vi "Discrete_TF_L_RT.vi"(10 "Gain":sgl, 11 "Input":sgl format="%#_13g") -> (3 "Output":sgl)   [LabVIEW 2019]
panel:
  in  "Numerator":sgl=5.6754 format="%#_13g"
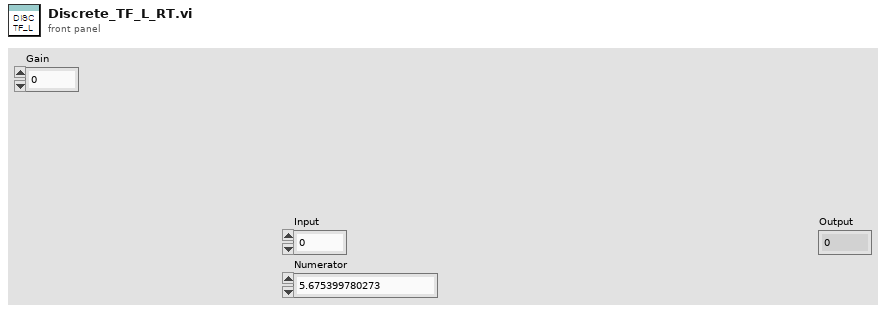
[diagram p1: front panel]
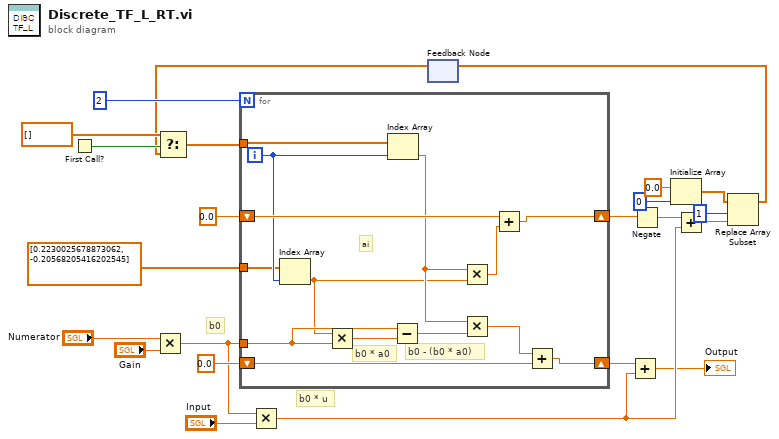
[diagram p0: block diagram]
diagram:
  # "b0"
  # "b0 * u"
  n1 = First Call?() -> (First Call?: T/F=w18:bool)
  n2 = Multiply(x="Numerator", y="Gain") -> (x*y=w9:sgl)
  n3 = Multiply(x=w9, y="Input") -> (x*y=w14:sgl)
  n4 = feedback #1() -> (w11:sgl[])  [unwired: 1 in]
  n5 = Select(t=sgl[] [], s=w18, f=w11) -> (s? t:f=w12:sgl[])
  n6 = for {
    N: 2 -> [_]
    tunnel: w9 -> [w36]
    shift-right: [w32] -> w21
    shift-left: sgl 0.0 -> [w33]
    shift-right: [w29] -> w16
    shift-left: sgl 0.0 -> [w30]
    tunnel: w12 -> [w28]
    tunnel: sgl[] [0.22300257, -0.20568205] ("배열") -> [w25]
    i -> [w26]
    # "b0 - (b0 * a0)"
    # "ai"
    # "b0 * a0"
    n7 = Index Array(array=w25, index=w26) -> (element=w24:sgl)
    n8 = Multiply(x=w24, y=w36) -> (x*y=w37:sgl)
    n9 = Index Array(array=w28, index=w26) -> (element=w27:sgl)
    n10 = Subtract(x=w36, y=w37) -> (x-y=w35:sgl)
    n11 = Multiply(x=w27, y=w24) -> (x*y=w31:sgl)
    n12 = Multiply(x=w27, y=w35) -> (x*y=w34:sgl)
    n13 = Add(x=w30, y=w31) -> (x+y=w29:sgl)
    n14 = Add(x=w34, y=w33) -> (x+y=w32:sgl)
  }
  n15 = Add(x=w21, y=w14) -> (x+y=→"Output":sgl)
  n16 = Negate(x=w16) -> (-x=w15:sgl)
  n17 = Initialize Array(sgl 0.0 ("원소"), 0 ("차원 크기")) -> (w5:sgl[])
  n18 = Add(x=w15, y=w14) -> (x+y=w3:sgl)
  n19 = Replace Array Subset(array=w5, new element=w3, index=1 ("인덱스")) -> (w2:sgl[])
  n20 = feedback-in #1(w2) -> ()
